vi "Day 21-Create Dice Sum Possibility Map.vi"() -> (3 "Map":map{u64, u64}(c390))   [LabVIEW 2021]
uses:
  <vilib>/Utility/miscctls.llb/LVMapReplaceAction.ctl
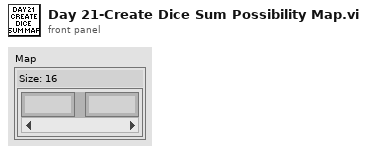
[diagram p1: front panel]
types:
  T1 = typedef "LVMapReplaceAction.ctl" = enum32{"Modify Entry only if found", "Add or Modify Entry", "Delete Entry"}
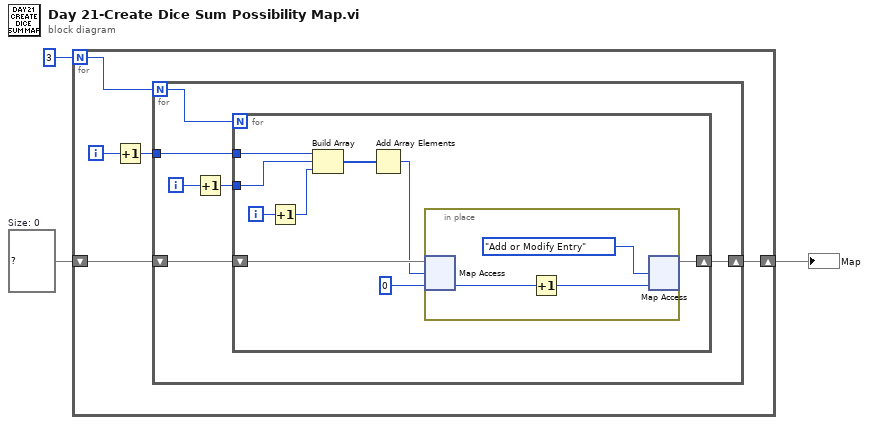
[diagram p0: block diagram]
diagram:
  w2 = map{u64, u64} {}  # Size: 0
  n1 = for {
    N: 3 -> [w6]
    shift-right: [w5] -> w3
    shift-left: w2 -> [w4]
    i -> [w8]
    n2 = Increment(x=w8) -> (x+1=w7:i32)
    n3 = for {
      N: w6 -> [w11]
      tunnel: w7 -> [w14]
      shift-right: [w10] -> w5
      shift-left: w4 -> [w9]
      i -> [w13]
      n4 = Increment(x=w13) -> (x+1=w12:i32)
      n5 = for {
        N: w11 -> [_]
        tunnel: w14 -> [w23]
        tunnel: w12 -> [w22]
        shift-right: [w16] -> w10
        shift-left: w9 -> [w19]
        i -> [w21]
        n6 = Increment(x=w21) -> (x+1=w20:i32)
        n7 = Build Array(w23, w22, w20) -> (w15:i32[])
        n8 = Add Array Elements(numeric array=w15) -> (sum=w18:i32)
        n9 = in-place {
          n10 = in-place-map #1(w19, w18, u64 0) -> (w26:u64)  [unwired: 1 out]
          n11 = Increment(x=w26) -> (x+1=w24:u64)
          n12 = in-place-map #1(w24, LVMapReplaceAction."Add or Modify Entry" ("action")) -> (w16:map{u64, u64})  [unwired: 2 out]
        }
      }
    }
  }
  "Map" <- w3
